vi "LauncherSystem.vi"() -> ()   [LabVIEW 2025]
panel:
  out "Intake RPM":dbl format="%12.1f"
  out "Intake Motor Dmd":dbl format="%11.2f"
  out "Position Deg":dbl format="%12.1f"
  out "Intake On":bool
  out "Down":bool
  # "INTAKE"
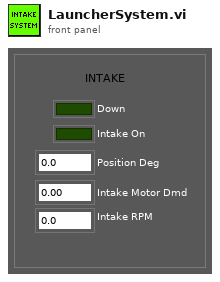
[diagram p1: front panel]
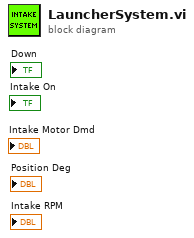
[diagram p0: block diagram]
diagram:
